vi "Simple Bluetooth - Client.vi"() -> ()   [LabVIEW 2016]
doc: "Demonstrates how to open a connection to a specified Bluetooth server and channel, read the data being sent to the channel, and display the data on a chart. This VI is designed to stop if the Bluetooth connection is terminated."
panel:
  in  "Server Closed":string="The server VI closed the connection."
  out "Waveform Graph":dbl[](graph)
  in  "Stop":bool
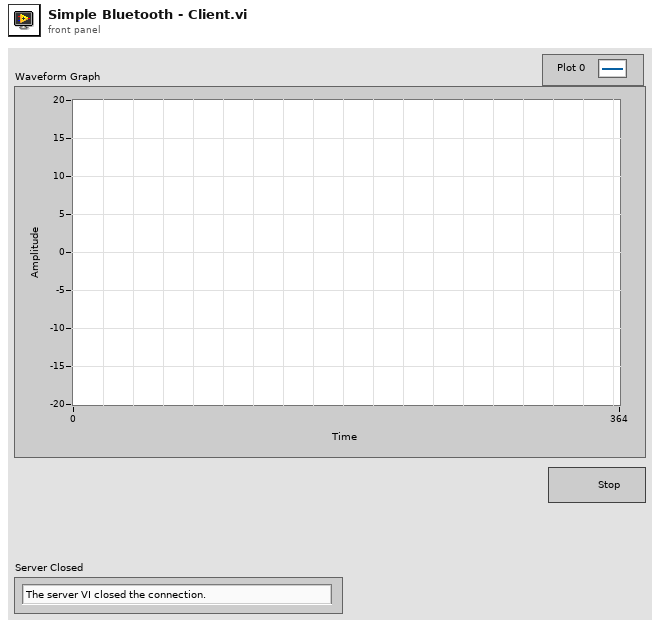
[diagram p1: front panel]
types:
  T1 = cluster{"Address":string, "Device Name":string}[]
  T2 = cluster{"channel":u16, "uuid":string, "service name":string, "service description":string}[]
  T3 = cluster{"channel":u16, "uuid":string, "service name":string, "service description":string}
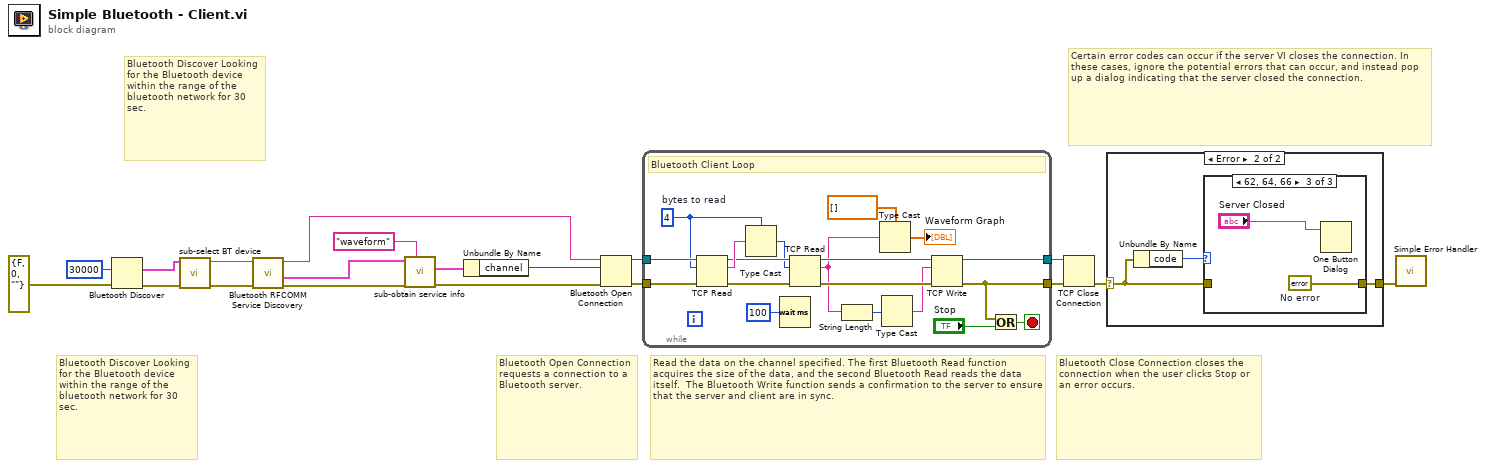
[diagram p0: block diagram]
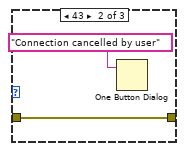
[diagram p4: hidden frame]
diagram:
  # "Bluetooth Discover Looking for the Bluetooth device within the range of the bluetooth network for 30 sec."
  # "Bluetooth Discover Looking for the Bluetooth device within the range of the bluetooth network for 30 sec."
  # "Certain error codes can occur if the server VI closes the connection. In these cases, ignore the potential errors that can occur, and instead pop up a dialog indicating that the server closed the connection."
  # "Bluetooth Close Connection closes the connection when the user clicks Stop or an error occurs."
  # "Read the data on the channel specified. The first Bluetooth Read function acquires the size of the data, and the second Bluetooth Read reads the data itself.  The Bluetooth Write function sends a confirmation to the server to ensure that the server and client are in sync."
  # "Bluetooth Open Connection requests a connection to a Bluetooth server."
  n1 = Bluetooth Discover(8:errorcluster {"status"=FALSE, "code"=0, "source"=""} ("error constant"), 10:30000 ("time limit ms (10000)")) -> (0:w7:errorcluster, 2:w12:T1)  [unwired: 1 out]
  n2 = call "sub-select BT device.vi"("error in (no error)"=w7, "device list"=w12) -> ("error out"=w9:errorcluster, "Address"=w3:string)  [unwired: 7 in, 1 out]
  n3 = call <vilib>:"Bluetooth RFCOMM Service Discovery.vi"("error in (no error)"=w9, "address in"=w3) -> ("error out"=w10:errorcluster, "service list"=w11:T2, "address out"=w1:string)  [unwired: 2 in, 1 out]
  n4 = call "sub-obtain service info.vi"("Service Name"="waveform", "error in (no error)"=w10, "service list"=w11) -> ("error out"=w6:errorcluster, "Service Info"=w5:T3)  [unwired: 7 in]
  n5 = Unbundle By Name(w5) -> ("channel"=w4:u16)
  n6 = Bluetooth Open Connection(8:w6, 10:w4, 11:w1) -> (0:w16:errorcluster, 3:w17:refnum<k31>)  [unwired: 2 in]
  n7 = while {
    tunnel: w16 -> [w33]
    tunnel: w17 -> [w34]
    tunnel: [w26] -> w18
    tunnel: [w21] -> w19
    stop <- w31 stop-if-true
    w20 = 4  # bytes to read
    # "Bluetooth Client Loop"
    n8 = TCP Read(connection ID=w34, bytes to read=w20, error in (no error)=w33) -> (connection ID out=w37:refnum<k31>, data out=w38:string, error out=w36:errorcluster)  [unwired: 2 in]
    n9 = Type Cast(type=w20, x=w38) -> (*(type *) &x=w35:i32)
    n10 = Wait (ms)(milliseconds to wait=u32 100) -> ()  [unwired: 1 out]
    n11 = TCP Read(connection ID=w37, bytes to read=w35, error in (no error)=w36) -> (connection ID out=w27:refnum<k31>, data out=w24:string, error out=w25:errorcluster)  [unwired: 2 in]
    n12 = String Length(string=w24) -> (length=w23:i32)
    n13 = Type Cast(type=dbl[] [] ("chart"), x=w24) -> (*(type *) &x=→"Waveform Graph":dbl[])
    n14 = Type Cast(x=w23) -> (*(type *) &x=w22:string)  [unwired: 1 in]
    n15 = TCP Write(connection ID=w27, data in=w22, error in (no error)=w25) -> (connection ID out=w26:refnum<k31>, error out=w21:errorcluster)  [unwired: 1 in, 1 out]
    n16 = Or(x=w21, y="Stop") -> (x .or. y?=w31:bool)
  }
  n17 = TCP Close Connection(connection ID=w18, error in (no error)=w19) -> (error out=w15:errorcluster)  [unwired: 1 in, 1 out]
  n18 = case shown="Error" w15 {
    selector: w15 -> [w39 w41]
    tunnel: [w39 w40] -> w14
    frame No Error {
    }
    frame Error {
      n19 = Unbundle By Name(w41) -> ("code"=w42:i32)
      n20 = case shown="62, 64, 66" w42 {
        tunnel: w41 -> [w43 w44 _]
        tunnel: [w43 w44 w47] -> w40
        frame Default {
        }
        frame 43 {
          n21 = One Button Dialog(message="Connection cancelled by user") -> ()  [unwired: 1 in, 1 out]
        }
        frame 62, 64, 66 {
          w47 = errorcluster {"status"=FALSE, "code"=0, "source"=""}  # No error
          n22 = One Button Dialog(message="Server Closed") -> ()  [unwired: 1 in, 1 out]
        }
      }
    }
  }
  n23 = call <vilib>:"Simple Error Handler.vi"("error in (no error)"=w14) -> ()  [unwired: 4 in, 5 out]
